vi "FA_PluginRef.vi"(8 "Error In":errorcluster) -> (0 "Error Out":errorcluster)   [LabVIEW 2014, in "FA_ApplySysConfig.lvlib"]
uses:
  FA_ApplySysConfig.lvlib
panel:
  # "This VI will likely be deleted once I have plugins to work with"
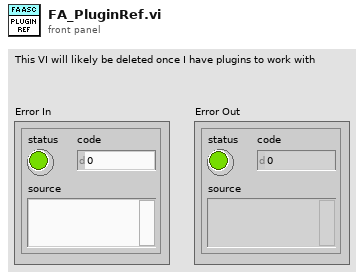
[diagram p1: front panel]
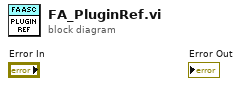
[diagram p0: block diagram]
diagram:
